vi "Flip Transform-Matrix Handedness.vi"(1 "4x4 Transform Matrix":T1) -> (0 "Flipped Handedness Transform Matrix":T1)   [LabVIEW 2020, in "ar.lvlib"]
doc: "Flip the Handedness of a 4x4 Transform Matrix between Left and Right or Right and Left Handedness."
uses:
  ar.lvlib
  <vilib>/Analysis/Matrix/Datatypes/RealMatrix.ctl
  <vilib>/Analysis/baseanly.llb/Real A x B.vi
  <vilib>/Analysis/NI_AALBase.lvlib
  <vilib>/Analysis/Matrix/NI_Matrix.lvlib
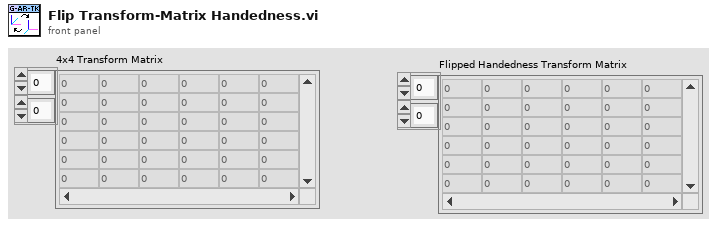
[diagram p1: front panel]
types:
  T1 = typedef "NI_Matrix.lvlib/RealMatrix.ctl" = dbl[][]
  T2 = typedef "ar.lvlib/tvec.ctl" = cluster{"x":dbl, "y":dbl, "z":dbl}
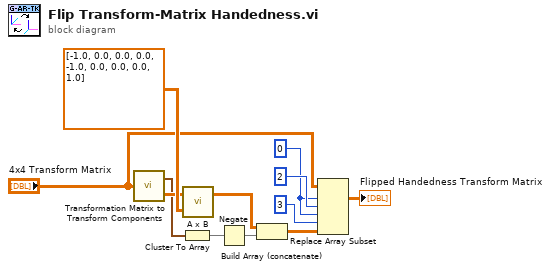
[diagram p0: block diagram]
diagram:
  w6 = 0 ("row 1")
  n1 = call "Transformation Matrix to Transform Components.vi"("4x4 Transformation Matrix"="4x4 Transform Matrix") -> ("tvec"=w2:T2, "Rotation Matrix"=w3:T1)
  n2 = Cluster To Array(cluster=w2) -> (array=w1:dbl[])
  n3 = call-poly <vilib>:"A x B.vi"("B"=T1 [[-1.0, 0.0, 0.0], [0.0, -1.0, 0.0], [0.0, 0.0, 1.0]], "A"=w3) -> ("A x B"=w12:T1)  [unwired: 1 out]
  n4 = Negate(x=w1) -> (-x=w10:dbl[])
  n5 = Build Array (concatenate)(w12, w10) -> (w9:T1)
  n6 = Replace Array Subset(array="4x4 Transform Matrix", new element=w9, index (dim 0)=w6, index (dim 1)=2 ("row N"), index (dim 2)=w6, index (dim 3)=3 ("column N")) -> (→"Flipped Handedness Transform Matrix":T1)
